vi "isHEXDigit.vi"(11 "characters":string) -> (3 "HEX Digits":bool)   [LabVIEW 2013, in "openURI.lvlib"]
uses:
  openURI.lvlib
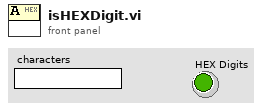
[diagram p1: front panel]
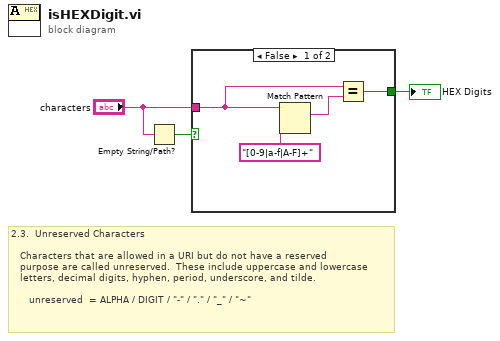
[diagram p0: block diagram]
diagram:
  # "2.3.  Unreserved Characters\n\n   Characters that are allowed in a URI but do not have a reserved\n   purpose are called unreserved.  These include uppercase and lowercase\n   letters, decimal digits, hyphen, period, underscore, and tilde.\n\n      unreserved  = ALPHA / DIGIT / \"-\" / \".\" / \"_\" / \"~\""
  n1 = Empty String/Path?(string/path="characters") -> (empty?=w3:bool)
  n2 = case shown="False" w3 {
    selector: w3 -> [_ w8]
    tunnel: "characters" -> [w6 _]
    tunnel: [w5 w8] -> w1
    frame False {
      n3 = Match Pattern(string=w6, regular expression="[0-9|a-f|A-F]+") -> (match substring=w7:string)  [unwired: 1 in, 3 out]
      n4 = Equal?(x=w6, y=w7) -> (x = y?=w5:bool)
    }
    frame True {
    }
  }
  "HEX Digits" <- w1
